vi "fgpa_close.vi"(8 "error in":errorcluster, 11 "FPGA VI Reference In":T1) -> (0 "error out":errorcluster)   [LabVIEW 2011, in "Fiberscope_library.lvlib"]
uses:
  Fiberscope_library.lvlib
  typedefs/fpga_main_spiral_fpga_ref.ctl
  <vilib>/FPGAPlugInAG/PXI-7813R/niLvFpga_Close_PXI-7813R.vi
  <vilib>/rvi/interface/nirviCloseFPGA/nirviCloseFPGA.xnode
  FPGA Bitfiles/FiberscopeRK1107_FPGATarget_fpgamainspiral_0DF2A7CB.lvbitx
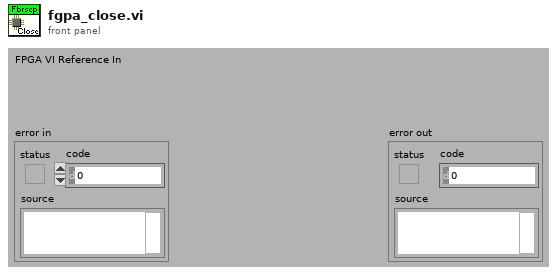
[diagram p1: front panel]
types:
  T1 = typedef "Fiberscope_library.lvlib/fpga_main_spiral_fpga_ref.ctl" = refnum<k20>
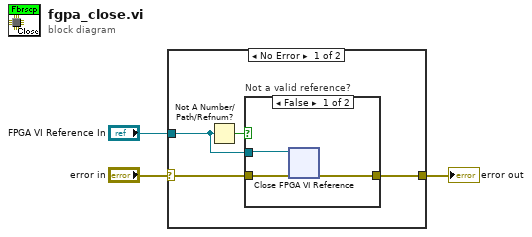
[diagram p0: block diagram]
diagram:
  n1 = case shown="No Error" "error in" {
    selector: "error in" -> [w6 w12]
    tunnel: [w5 w12] -> w2
    tunnel: "FPGA VI Reference In" -> [w4 _]
    frame No Error {
      n2 = Not A Number/Path/Refnum?(number/path/refnum=w4) -> (NaN/Path/Refnum?=w7:bool)
      n3 = case "Not a valid reference?" shown="False" w7 {
        tunnel: w6 -> [w10 w11]
        tunnel: [w9 w11] -> w5
        tunnel: w4 -> [w8 _]
        frame False {
          n4 = xnode "Close FPGA VI Reference"("FPGA VI Reference In"=w8, "error in"=w10) -> ("error out"=w9:errorcluster)
        }
        frame True {
        }
      }
    }
    frame Error {
    }
  }
  "error out" <- w2
